vi "FP-Version.vi"() -> (0 "FP Version":string)   [LabVIEW 2019]
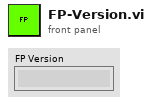
[diagram p1: front panel]
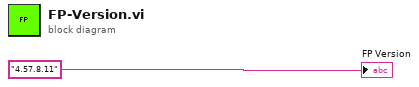
[diagram p0: block diagram]
diagram:
  "FP Version" <- "4.57.8.11"
